vi "Show FPGA Map.vi"() -> ()   [LabVIEW 2012]
uses:
  Type/_RT Command.ctl
panel:
  in  "Map Type:":u16(ring) items=["Method", "Q1 Cal +", "Q2 Cal +", "Q1 Cal -", "Q2 Cal -", "Q1 Res Hi +", "Q2 Res Hi +", "Q1 Res Med +", "Q2 Res Med +", "Q1 Res Lo +", "Q2 Res Lo +", "Q1 Res Hi -", "Q2 Res Hi -", "Q1 Res Med -", "Q2 Res Med -", "Q1 Res Lo -", "Q2 Res Lo -"]
  out "Listbox":i32(listbox)
  in  "Done":bool
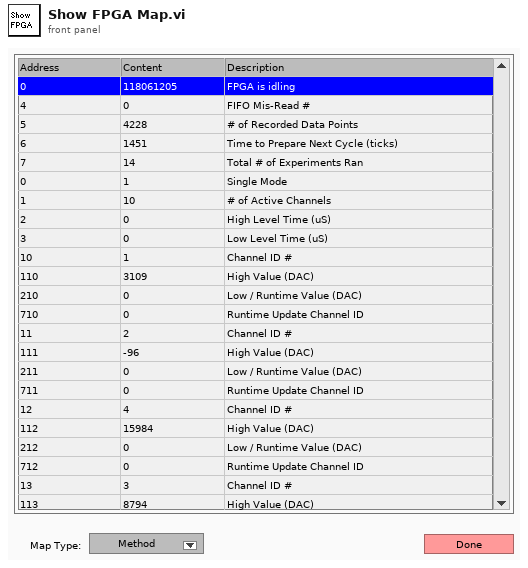
[diagram p1: front panel]
types:
  T1 = typedef "_RT Command.ctl" = enum16{"Start", "Stop", "Runtime Update", "Get Data", "Get Info", "Get Status", "Get Param", "Get Config", "Get Table", "Read ADC", "Set Oscillator", "Update Config", "Update Table", "Set All Pol", "Set Pol and DC", "Set Max Mass", "Toggle RP", "Toggle EL", "Set PIC", "Initialize Turbo", "Send Turbo Comm", "Close Turbo", "P1", "P2", "P3", "Send Serial", "Set LC Out", "Get LC In", "Read VAC", "Test Table", "Toggle Power", "Get Startup", "Set Startup", "Get ADC Table", "Set ADC Table", "Get Brief Status", "Get Detail Status", "Auxiliary Update", "Set CC Logics", "Set CC Input Logics", "Ignore Error"}
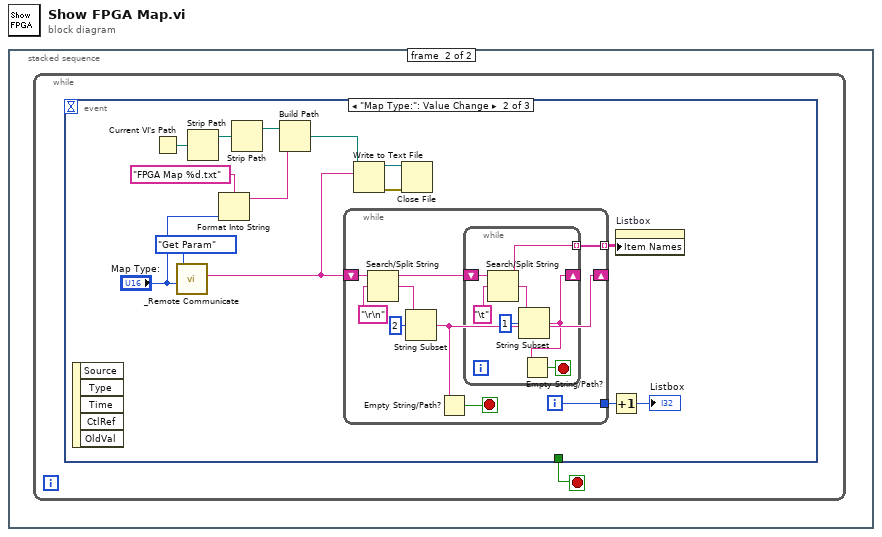
[diagram p0: block diagram]
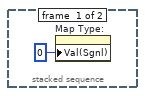
[diagram p2: hidden frame]
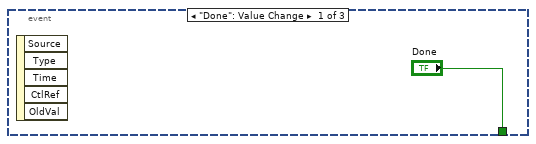
[diagram p3: hidden frame]
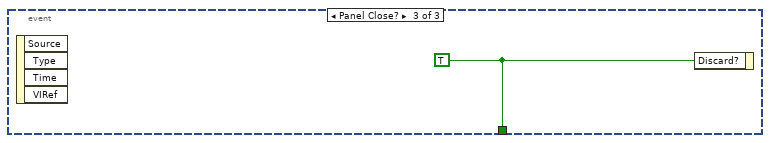
[diagram p4: hidden frame]
diagram:
  n1 = stacked-sequence {
    frame #0 {
      n2 = property on="Map Type:" class="Ring (strict)"("Val(Sgnl)"=u16 0 ("Value (Signaling)")) -> ()  [unwired: 2 in, 2 out]
    }
    frame #1 {
      n3 = while {
        stop <- w2 stop-if-true
        n4 = event shown="[1] \"Map Type:\": Value Change" {
          selector: _ -> [_ _ _]
          dyn-events: _ -> [_ _ _]
          timeout: _ -> [_ _ _]
          tunnel: ["Done" _ w34] -> w2
          event "Done": Value Change {
            n5 = event-data() -> ()  [unwired: 6 out]
          }
          event "Map Type:": Value Change {
            n6 = event-data() -> ()  [unwired: 6 out]
            n7 = Current VI's Path() -> (path=w12:path)
            n8 = call "_Remote Communicate.vi"("DC Param"="Map Type:", "Command"=_RT_Command."Get Param") -> ("Info"=w6:string)  [unwired: 4 in, 3 out]
            n9 = Strip Path(path=w12) -> (stripped path=w13:path)  [unwired: 1 out]
            n10 = Format Into String(format string="FPGA Map %d.txt", "Map Type:") -> (resulting string=w7:string)  [unwired: 2 in, 1 out]
            n11 = Strip Path(path=w13) -> (stripped path=w14:path)  [unwired: 1 out]
            n12 = Build Path(base path=w14, name or relative path=w7) -> (appended path=w11:path)
            n13 = while {
              shift-right: [w19] -> _
              shift-left: w6 -> [w26]
              tunnel: [w21] -> w17 mode=indexing
              tunnel: [w18] -> w15
              i -> [w18]
              stop <- w20 stop-if-true
              n14 = Search/Split String(string=w26, search string/char (-)="\r\n") -> (substring before match=w22:string, match + rest of string=w24:string)  [unwired: 2 out]
              n15 = String Subset(string=w24, offset (0)=2) -> (substring=w19:string)  [unwired: 1 out]
              n16 = Empty String/Path?(string/path=w19) -> (empty?=w20:bool)
              n17 = while {
                shift-right: [w27] -> _
                shift-left: w22 -> [w32]
                tunnel: [w31] -> w21 mode=indexing
                stop <- w28 stop-if-true
                n18 = Search/Split String(string=w32, search string/char (-)="\t") -> (substring before match=w31:string, match + rest of string=w29:string)  [unwired: 2 out]
                n19 = String Subset(string=w29, offset (0)=1) -> (substring=w27:string)  [unwired: 1 out]
                n20 = Empty String/Path?(string/path=w27) -> (empty?=w28:bool)
              }
            }
            n21 = Write to Text File(file (use dialog)=w11, text=w6) -> (refnum out=w4:refnum<file>, error out=w5:errorcluster)  [unwired: 2 in, 1 out]
            n22 = Close File(refnum=w4, error in=w5) -> ()  [unwired: 2 out]
            n23 = Increment(x=w15) -> (x+1=→"Listbox":i32)
            n24 = property on="Listbox" class="MCListbox (strict)"("Item Names"=w17) -> ()  [unwired: 2 in, 2 out]
          }
          event Panel Close? {
            w34 = TRUE ("Discard?")
            n25 = event-data() -> ()  [unwired: 5 out]
            n26 = event-data("Discard?"=w34) -> ()  [unwired: 1 in, 1 out]
          }
        }
      }
    }
  }
